vi "InsertHistogramIndices.vi"(0 "Insert index":i32, 1 "Rising flank?":bool, 5 "Histogram indices":i32[](array[numeric])=[0, 0, 0, 0, 0, 0, 0, 0, 0, 0], 7 "Master array in":i32[](array[numeric])=[0, 0, 0, 0, 0, 0, 0, 0, 0, 0, 0, 0, 0, 0, 0, 0, 0, 0, 0, 0, 0, 0, 0, 0, 0, 0, 0, 0, 0, 0, 0, 0, 0, 0, 0, 0, 0, 0, 0, 0, 0, 0, 0, 0, 0, 0, 0, 0, 0, 0, 0, 0, 0, 0, 0, 0, 0, 0, 0, 0]) -> (8 "Master array out":i32[](array[numeric]))   [LabVIEW 2012]
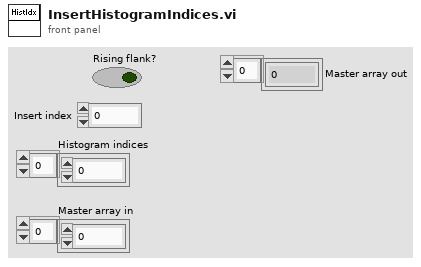
[diagram p1: front panel]
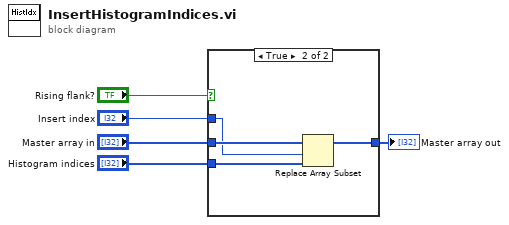
[diagram p0: block diagram]
diagram:
  n1 = case shown="True" "Rising flank?" {
    tunnel: "Histogram indices" -> [_ w10]
    tunnel: "Master array in" -> [w6 w9]
    tunnel: "Insert index" -> [_ w8]
    tunnel: [w6 w7] -> w1
    frame False {
    }
    frame True {
      n2 = Replace Array Subset(array=w9, new element=w10, index=w8) -> (w7:i32[])
    }
  }
  "Master array out" <- w1
